vi "serial.vi"() -> ()   [LabVIEW 2020]
uses:
  <vilib>/Instr/_visa.llb/VISA Configure Serial Port (Instr).vi
panel:
  out "concatenated string":string
  in  "Button":bool
  in  "Stop":bool
  out "error out":errorcluster
  in  "VISA resource name":refnum<visa-resource-name>
  in  "Array":cluster{"x":dbl, "y":dbl}[](array[cluster])
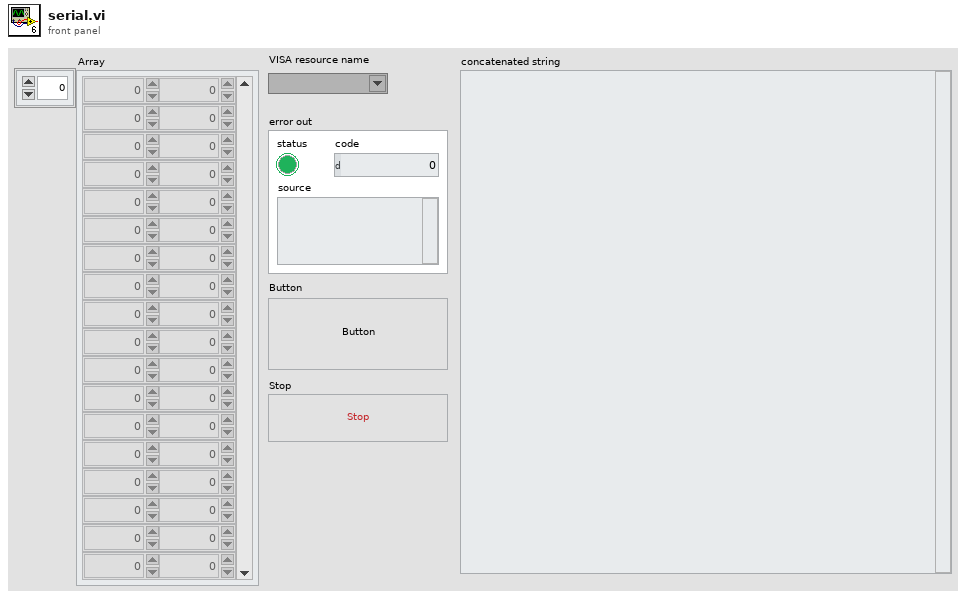
[diagram p1: front panel]
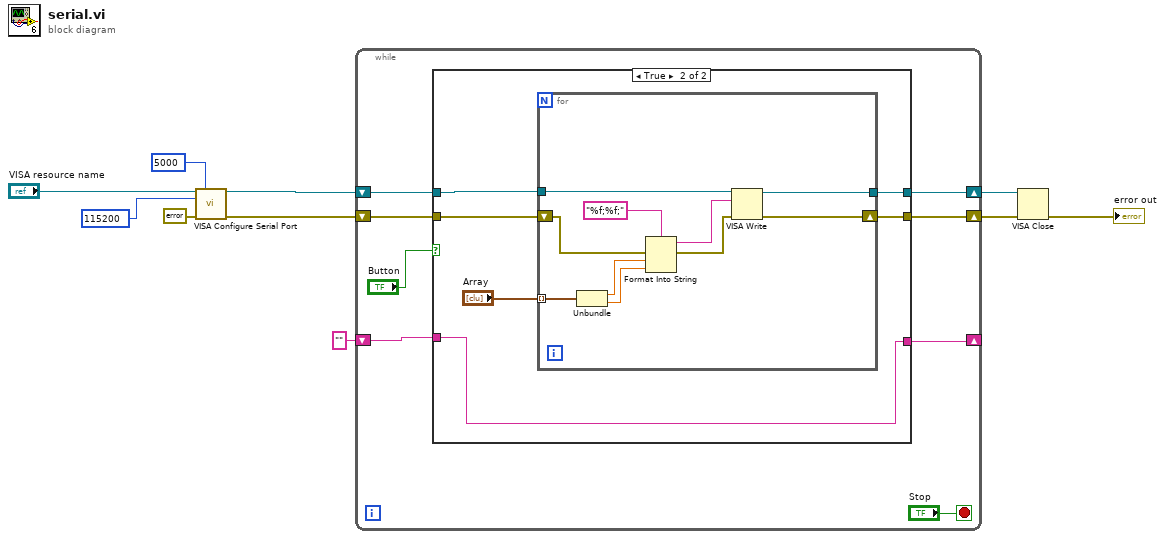
[diagram p0: block diagram]
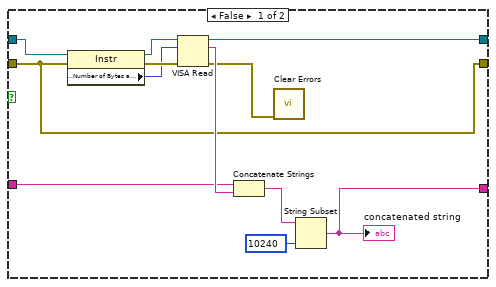
[diagram p2: hidden frame]
diagram:
  n1 = call-poly "VISA Configure Serial Port"("VISA resource name"="VISA resource name", "timeout (10sec)"=u32 5000, "baud rate (9600)"=u32 115200, "error in (no error)"=errorcluster {"status"=FALSE, "code"=0, "source"=""}) -> ("VISA resource name out"=w5:refnum<visa-resource-name>, "error out"=w6:errorcluster)  [unwired: 10 in]
  n2 = while {
    shift-right: [w16] -> w4
    shift-left: w6 -> [w18]
    shift-right: [w15] -> w3
    shift-left: w5 -> [w17]
    shift-right: [w12] -> _
    shift-left: "" -> [w11]
    stop <- "Stop" stop-if-true
    n3 = case shown="True" "Button" {
      tunnel: w18 -> [w22 w36]
      tunnel: w17 -> [w30 w34]
      tunnel: [w22 w33] -> w16
      tunnel: [w26 w32] -> w15
      tunnel: [w20 w31] -> w12
      tunnel: w11 -> [w24 w31]
      frame False {
        n4 = property class="Instr"(reference=w30, error in=w22) -> (reference out=w28:refnum<visa-resource-name>, error out=w29:errorcluster, "Serial Settings:Number of Bytes at Serial Port"=w27:u32)
        n5 = VISA Read(VISA resource name=w28, byte count=w27, error in (no error)=w29) -> (VISA resource name out=w26:refnum<visa-resource-name>, read buffer=w25:string, error out=w23:errorcluster)  [unwired: 1 out]
        n6 = Concatenate Strings(w24, w25) -> (w21:string)
        n7 = call <vilib>:"Clear Errors.vi"("error in (no error)"=w23) -> ()  [unwired: 5 in, 2 out]
        n8 = String Subset(string=w21, length (rest)=10240 ("length (rest)")) -> (substring=w20:string)  [unwired: 1 in]
        "concatenated string" <- w20
      }
      frame True {
        n9 = for {
          shift-right: [w38] -> w33
          shift-left: w36 -> [w45]
          tunnel: "Array" -> [w43] mode=indexing
          tunnel: w34 -> [w46]
          tunnel: [w37] -> w32
          n10 = Unbundle(w43) -> ("x"=w42:dbl, "y"=w41:dbl)
          n11 = Format Into String(format string="%f;%f;", error in=w45, w42, w41) -> (resulting string=w39:string, error out=w40:errorcluster)  [unwired: 1 in]
          n12 = VISA Write(VISA resource name=w46, write buffer=w39, error in (no error)=w40) -> (VISA resource name out=w37:refnum<visa-resource-name>, error out=w38:errorcluster)  [unwired: 1 out]
        }
      }
    }
  }
  n13 = VISA Close(VISA resource name=w3, error in (no error)=w4) -> (error out=→"error out":errorcluster)
